vi "Wait on Event Sync.vi"(8 "error in (no error)":errorcluster, 9 "Module ID":u32) -> (0 "error out":errorcluster)   [LabVIEW 2014, in "GenNet-Server.lvlib"]
doc: "Wait on the rendezvous that synchronizes the registration of the events.\n_____\nBased on Delacor QMH Project Template 3.1.0.34."
uses:
  GenNet-Server.lvlib
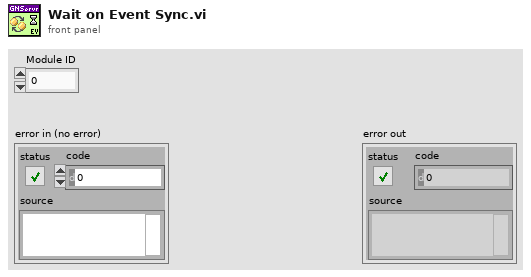
[diagram p1: front panel]
types:
  T1 = typedef "Rendezvous RefNum" = refnum<k1>
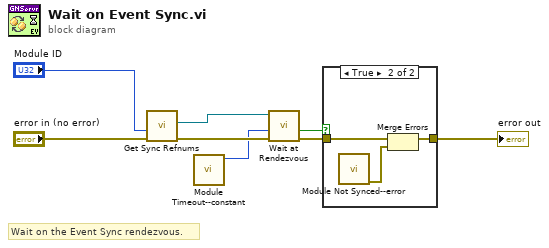
[diagram p0: block diagram]
diagram:
  # "Wait on the Event Sync rendezvous."
  n1 = call "Get Sync Refnums.vi"("error in (no error)"="error in (no error)", "Module ID"="Module ID") -> ("error out"=w7:errorcluster, "Event Sync"=w6:T1)  [unwired: 6 in, 2 out]
  n2 = call "Module Timeout--constant.vi"() -> ("Module Timeout"=w5:i32)  [unwired: 11 in]
  n3 = call <vilib>:"Wait at Rendezvous.vi"("error in (no error)"=w7, "ms timeout (-1)"=w5, "rendezvous"=w6) -> ("error out"=w3:errorcluster, "timed out"=w1:bool)  [unwired: 2 in, 1 out]
  n4 = case shown="True" w1 {
    tunnel: w3 -> [w9 w12]
    tunnel: [w9 w11] -> w2
    frame False {
    }
    frame True {
      n5 = call "Module Not Synced--error.vi"() -> ("error out"=w10:errorcluster)  [unwired: 11 in]
      n6 = Merge Errors(w12, w10) -> (w11:errorcluster)
    }
  }
  "error out" <- w2
